vi "ReadFailureRecordData_readFailureRecordParameters.vi"(8 "error in (no error)":errorcluster, 10 "failureRecordIdentifier":T1 {"DTCFailureType" format="%.0x"; "DTC ID" format="%.0x"; "failureRecordNumber" format="%.0x"}, 11 "diag ref in":T2) -> (0 "error out":errorcluster, 1 "success?":bool, 2 "data out":u8[](array[numeric]) format="%.0x", 3 "diag ref out":T2)   [LabVIEW 2013, in "GMLAN.lvlib"]
uses:
  GMLAN.lvlib
  <vilib>/Automotive Diagnostic Command Set/Diagnostic Transport.llb/Diag Reference.ctl
  <vilib>/Automotive Diagnostic Command Set/Diagnostic Transport.llb/Transport Protocol Selector.ctl
  <vilib>/Automotive Diagnostic Command Set/Diagnostic Transport.llb/Diag CAN Frame Log.ctl
  ReadFailureRecordData_readFailureRecordParameters_failureRecordIdentifier.ctl
  <vilib>/addons/Automotive Diagnostic Command Set/NI_Automotive Diagnostic Command Set.lvlib
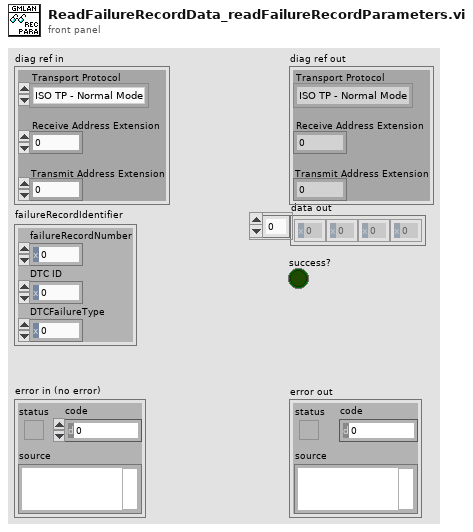
[diagram p1: front panel]
types:
  T1 = typedef "GMLAN.lvlib/ReadFailureRecordData_readFailureRecordParameters_failureRecordIdentifier.ctl" = cluster{"failureRecordNumber":u8, "DTC ID":u16, "DTCFailureType":u8}
  T2 = typedef "NI_Automotive Diagnostic Command Set.lvlib/Diag Reference.ctl" = cluster{"Diag CAN Handle":u32, "Transport Protocol":T3, "Receive Address Extension":u8, "Transmit Address Extension":u8, "Receive CAN Id":u32, "Transmit CAN Id":u32, "Diag CAN Queue":refnum<queue>, "Log Frames ?":bool, "My TP Address":u8, "Other TP Address":u8, "T1":u16, "T2":u16, "T3":u16, "T4":u16, "Tx SN":u8, "Block Size":u8, "Rx SN":u8, "VW TP Initialized?":bool, "Tx block no":u8, "baud rate":u32, "Interface":string, "Channel Diag CAN Handle":u32, "UDP Connection ID":refnum<k16>, "TCP Connection ID":refnum<k5>, "Target IP Addr":u32, "Source Address":u16, "Target Address":u16, "Send Header NACK?":bool, "DLL Handle":u32, "NAD":u8, "Time Stamp read first":dbl, "Time Stamp read last":dbl, "Time Stamp write first":dbl, "Time Stamp write last":dbl, "Time Stamp write":dbl, "Time Stamp read":dbl}
  T3 = typedef "NI_Automotive Diagnostic Command Set.lvlib/Transport Protocol Selector.ctl" = enum16{"ISO TP - Normal Mode", "ISO TP - Mixed Mode", "VW TP 2.0", "Diagnostics on IP", "ISO TP LIN"}
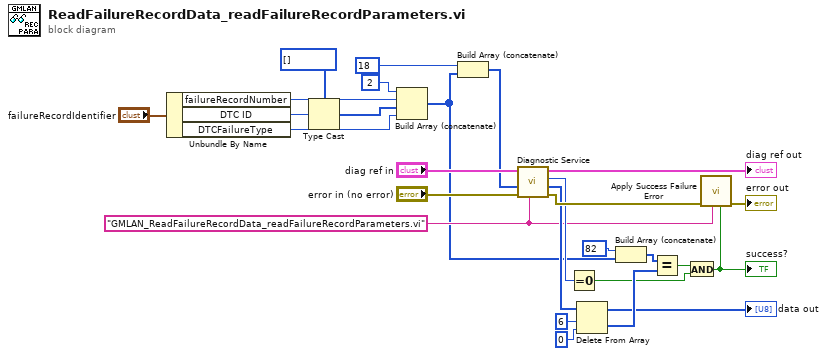
[diagram p0: block diagram]
diagram:
  w11 = "GMLAN_ReadFailureRecordData_readFailureRecordParameters.vi" ("error source")
  n1 = Unbundle By Name("failureRecordIdentifier") -> ("failureRecordNumber"=w8:u8, "DTC ID"=w6:u16, "DTCFailureType"=w7:u8)
  n2 = Type Cast(type=u8[] [], x=w6) -> (*(type *) &x=w4:u8[])
  n3 = Build Array (concatenate)(u8 2 ("element"), w8, w4, w7) -> (w2:u8[])
  n4 = Build Array (concatenate)(u8 18 ("element"), w2) -> (w1:u8[])
  n5 = call <vilib>:"Diagnostic Service.vi"("error source"=w11, "error in (no error)"="error in (no error)", "data in"=w1, "diag ref in"="diag ref in") -> ("error out"=w25:errorcluster, "data out"=w19:u8[], "error code"=w24:u8, "diag ref out"=→"diag ref out":T2)  [unwired: 2 in, 2 out]
  n6 = Equal To 0?(x=w24) -> (x = 0?=w17:bool)
  n7 = Delete From Array(array=w19, length=6, index=0) -> (deleted portion=w18:u8[], array with subset deleted=→"data out":u8[])
  n8 = Build Array (concatenate)(u8 82 ("element"), w2) -> (w20:u8[])
  n9 = Equal?(x=w20, y=w18) -> (x = y?=w15:bool)
  n10 = And(x=w15, y=w17) -> (x .and. y?=w12:bool)
  "success?" <- w12
  n11 = call <vilib>:"Apply Success Failure Error.vi"("success code"=w12, "error source"=w11, "error in (no error)"=w25) -> ("error out"=→"error out":errorcluster)  [unwired: 8 out]
